vi "Start GNU Octave.vi"(0 "working dir (user home)":path, 1 "full start timeout [ms] (20000)":u32=20000, 2 "Matlab script mode (F)":bool, 5 "octave binary file or dir (autofind)":path, 7 "path to lv_proc.dll (.)":path, 9 "hide debug console (T)":bool=TRUE, 11 "error in":errorcluster, 12 "wait for full start (T)":bool=TRUE, 13 "disable history (T)":bool=TRUE) -> (3 "GNU Octave version":string, 4 "GOLPI ref. out":T1={"pipe handle"={"lv_proc.dll file path"=path "", "process instance handle"=[], "debug mode"=FALSE, "debug data"=[]}, "fast read timeout [ms]"=500, "fast read settle time [ms]"=10, "fast read to multiple [ms]"=1, "max elements per input line"=100, "slow read timeout [ms]"=500, "stdin double format specifier"="", "max elements per stdout output column"=100, "console mode bitstream"=FALSE, "bitstream first read timeout [ms]"=1000, "bitstream read timeout [ms]"=50, "struct transfer possible"=FALSE, "matlab mode"=FALSE, "var pipe write timeout [ms]"=5000, "variable pipe mode"=FALSE, "variable pipe buffer size [Bytes]"=10000000, "variable pipe block size [Bytes]"=1000000} {"variable pipe block size [Bytes]" format="%.0p"; "variable pipe buffer size [Bytes]" format="%.0p"}, 14 "initial output":string, 15 "error out":errorcluster)   [LabVIEW 2020, in "GOLPI library.lvlib"]
doc: "Starts the GNU Octave.\nIf working directory is empty, VI sets it to user Documents directory.\n\nOctave binary file or directory is the executable file or directory containing the 'octave.bat' executable file (or 'octave-cli.exe', 'octave.exe'). Script .bat is prefered, because it sets libraries paths properly. If ommited, VI tries to find latest Octave installation.\n\nInitial output is the informations printed after start on the screen by GNU Octave. Set higher vlaue for 'Full start timeout' in the case GNU Octave loads a lot of packages.\n\nIf option 'Matlab script mode' is True, the VI will start Matlab using NI's Matlab script node. All followed VI calls of this library will then use Matlab instead of GNU Octave. That also means only used input option is 'wait fo full start'. Rest will be ignored.\n\nIf 'Wait for full start' is disabled, vi starts GNU Octave/Matlab and do not wait for the end of starting sequence. It is usefull if GNU Octave/Matlab loads a lot of packages at startup and the start can take several seconds. 'Version' and 'Initial output' is not returned. User can check himself if Octave finished starting sequence by waiting for keyword 'GOLPImarkstart' in the stdout (i.e. use 'Read Output Till Keyword.vi'). Note this is not supported for Matlab mode.\n\nSet 'hide window' to false to show console window (no effect in Matlab mode). Thus user can watch commands sent to GNU Octave and its output. Window is not interactive, only for debug purposes.\n\nIf 'Disable history' is set, all commands sent to GNU Octave will not be saved to GNU Octave history file. This is recommended especially when large data transfers are expected. This has no effect in Matlab mode.\n\n---\nGOLPI works only with 'lv_proc.dll' library in the GNU Octave mode, which is part of vipm package or should be delivered together with packed library. Placement of this dll is selected in terminal of Start GNU Octave.vi."
uses:
  GOLPI library.lvlib
  GOLPI reference Type Def.ctl
  LV Process source distribution/Pipe Handle.ctl
  <vilib>/Utility/sysdir.llb/System Directory Type.ctl
  Private/Type Definitions/Custom Error Codes Enum Type Def.vi
  <vilib>/regexp/Match Regular Expression.xnode
  LV Process source distribution/LV Process library.lvlib
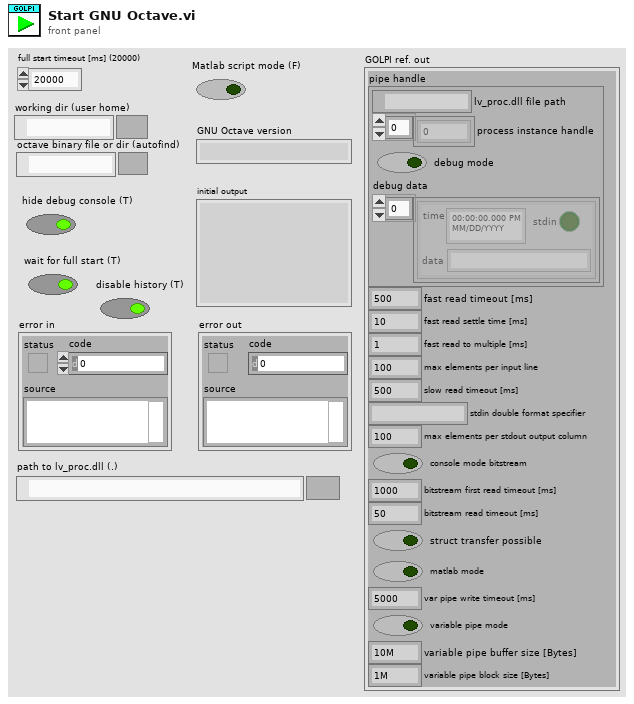
[diagram p1: front panel]
types:
  T1 = typedef "GOLPI library.lvlib/GOLPI reference Type Def.ctl" = cluster{"pipe handle":T2, "fast read timeout [ms]":u32, "fast read settle time [ms]":u32, "fast read to multiple [ms]":u32, "max elements per input line":u32, "slow read timeout [ms]":u32, "stdin double format specifier":string, "max elements per stdout output column":u32, "console mode bitstream":bool, "bitstream first read timeout [ms]":u32, "bitstream read timeout [ms]":u32, "struct transfer possible":bool, "matlab mode":bool, "var pipe write timeout [ms]":u32, "variable pipe mode":bool, "variable pipe buffer size [Bytes]":u32, "variable pipe block size [Bytes]":u32}
  T2 = typedef "LV Process library.lvlib/Pipe Handle.ctl" = cluster{"lv_proc.dll file path":path, "process instance handle":u32[], "debug mode":bool, "debug data":cluster{"time":timestamp, "stdin":bool, "data":string}[]}
  T3 = typedef "GOLPI library.lvlib/Custom Error Codes Enum Type Def.vi" = enum16{"no error", "00 working directory PAR1 missing", "01 octave binary PAR1 missing", "02 octave report error PAR1", "03 empty output last cmd PAR1", "04 missing temporary file PAR1", "05 pwd PAR 1 not exist", "06 oct package not installed", "07 octave default binary missing", "10 var PAR1 not string, vect", "11 var PAR1 not num, scal, ~compl", "12 var PAR1 not num, scal, compl", "13 var PAR1 not num, vect, ~compl", "14 var PAR1 not num, vect, compl", "15 var PAR1 not num, mat, ~compl", "16 var PAR1 not num, mat, ~compl", "30 read timeout", "60 bitstream transport failed", "61 bitstream decode error PAR1", "62 bitstream cannot be set", "70 struct transfer not possible", "80 struct: cluster elem. PAR1 not implem.", "81 struct: structure field PAR1 not implem.", "82 struct: size mismatch of PAR1", "83 struct: type mismatch of PAR1", "98 internal error", "99 not finished", "90 Not supported in Matlab mode", "91 Matlab variable transfer error", "92 Matlab Script Error", "100 Variable Pipe Mode cannot be set"}
  T4 = typedef "System Directory Type.ctl" = i32
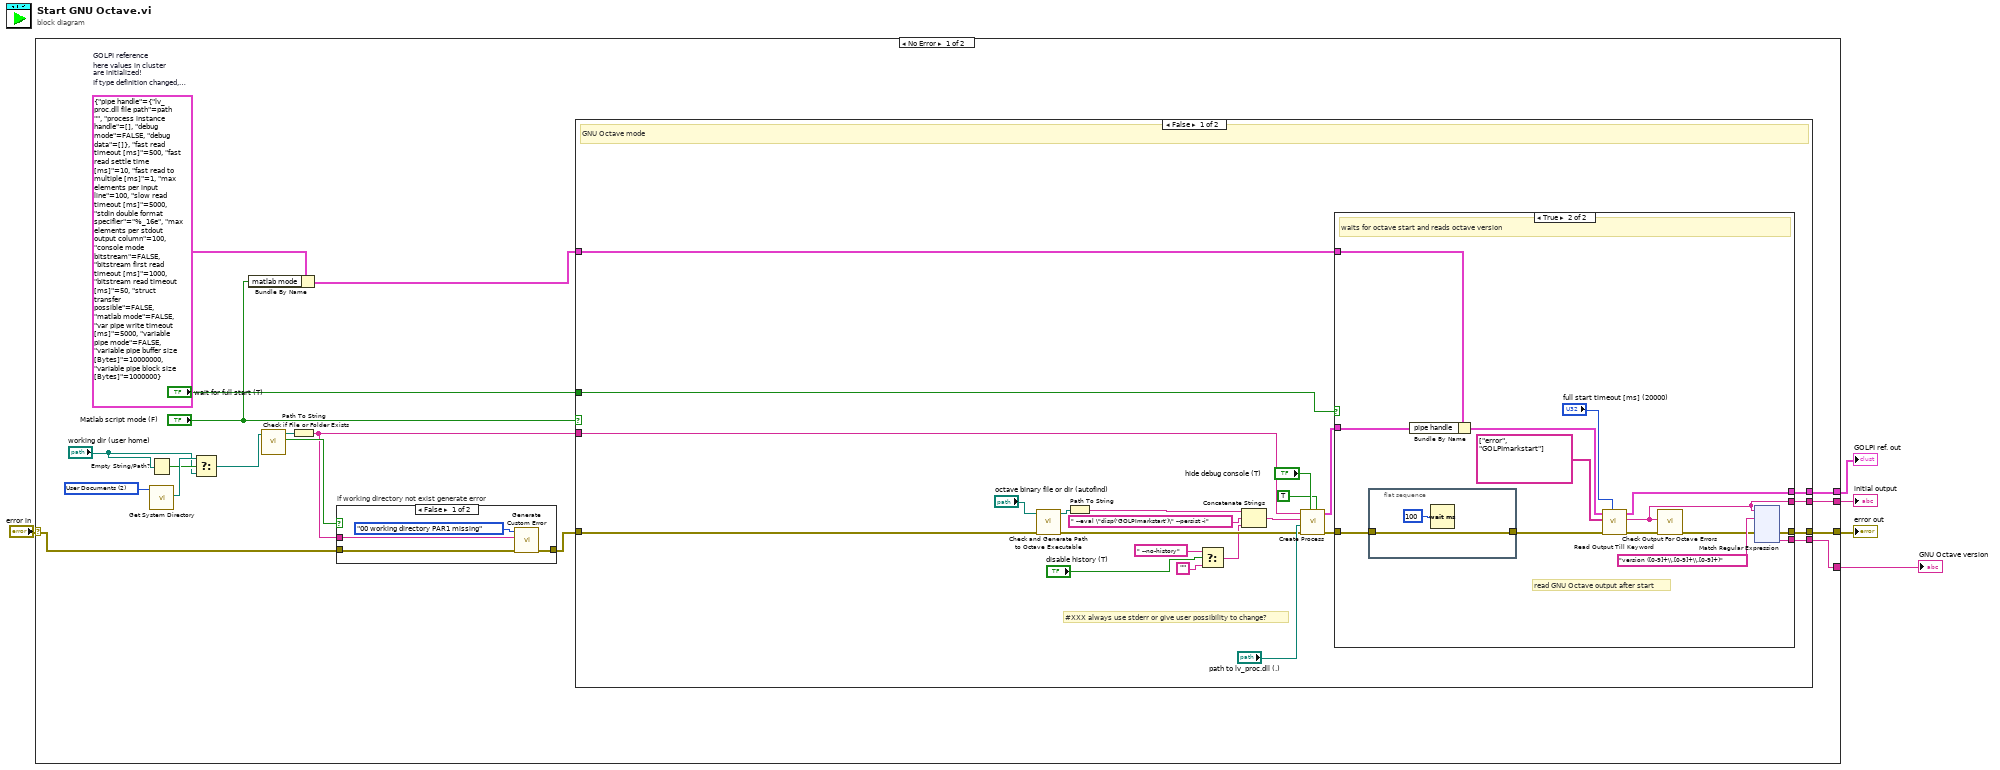
[diagram p0: block diagram]
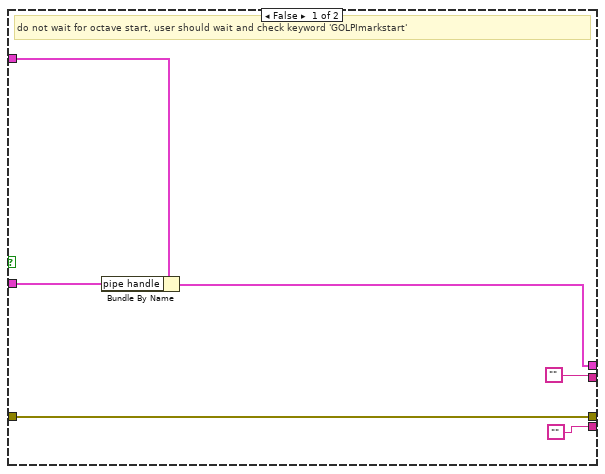
[diagram p3: hidden frame]
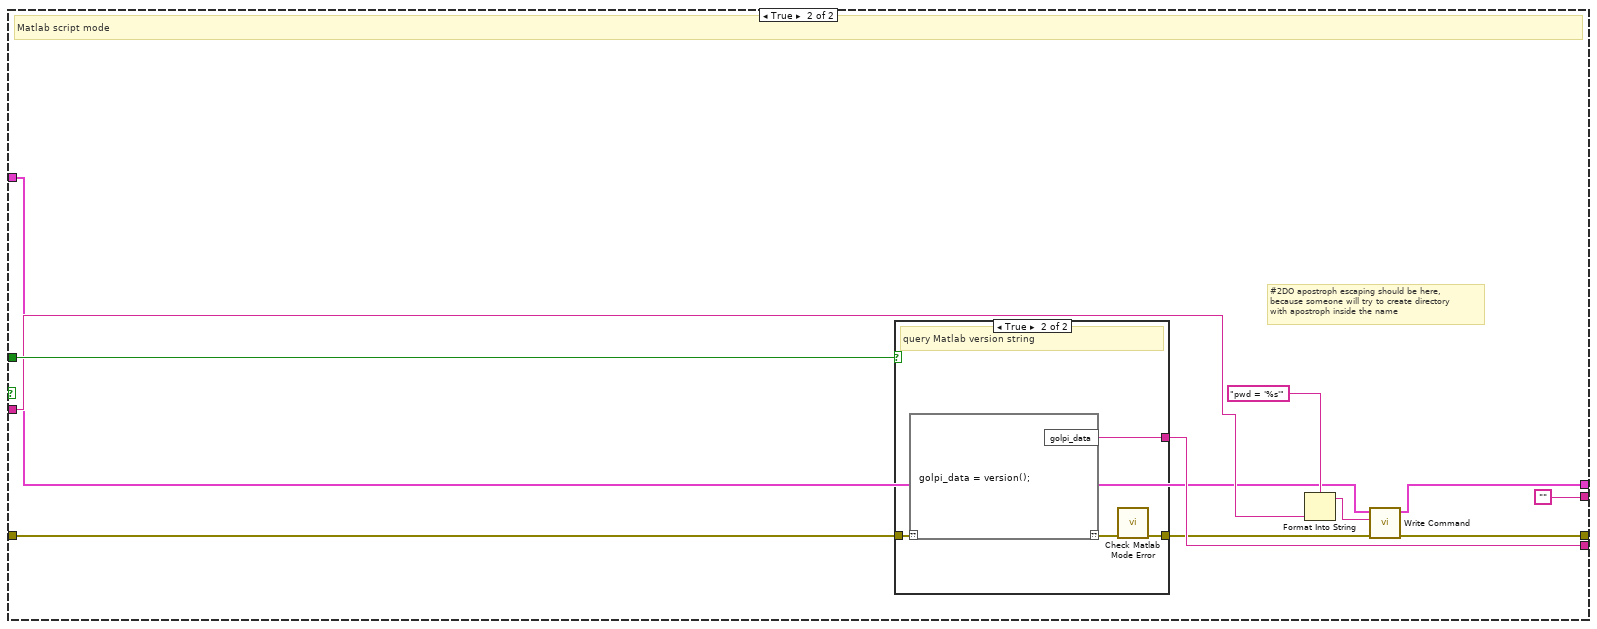
[diagram p4: hidden frame]
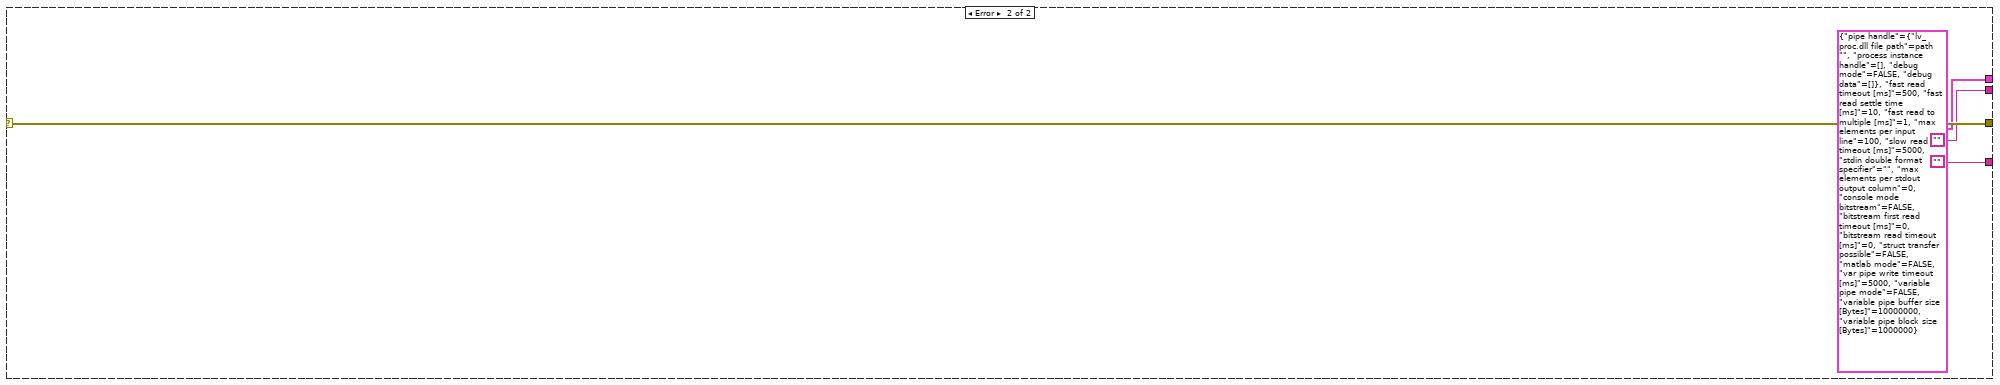
[diagram p6: hidden frame]
diagram:
  n1 = case shown="No Error" "error in" {
    selector: "error in" -> [w6 w209]
    tunnel: [w21 w209] -> w4
    tunnel: [w23 ""] -> w3
    tunnel: [w20 ""] -> w2
    tunnel: [w22 T1 {"pipe handle"={"lv_proc.dll file path"=path "", "process instance handle"=[], "debug mode"=FALSE, "debug data"=[]}, "fast read timeout [ms]"=500, "fast read settle time [ms]"=10, "fast read to multiple [ms]"=1, "max elements per input line"=100, "slow read timeout [ms]"=5000, "stdin double format specifier"="", "max elements per stdout output column"=0, "console mode bitstream"=FALSE, "bitstream first read timeout [ms]"=0, "bitstream read timeout [ms]"=0, "struct transfer possible"=FALSE, "matlab mode"=FALSE, "var pipe write timeout [ms]"=5000, "variable pipe mode"=FALSE, "variable pipe buffer size [Bytes]"=10000000, "variable pipe block size [Bytes]"=1000000} ("GOLPI ref.")] -> w1
    frame No Error {
      w15 = T4 2 items=["User Home"=0, "User Desktop"=1, "User Documents"=2, "User Application Data"=3, "User Preferences"=4, "User Temporary"=5, "Public Documents"=6, "Public Application Data"=7, "Public Preferences"=8, "Public Cache"=13, "System Core Libraries"=9, "System Installed Libraries"=10, "Application Files"=11, "Boot Volume Root"=12] ("system directory type")
      w18 = T1 {"pipe handle"={"lv_proc.dll file path"=path "", "process instance handle"=[], "debug mode"=FALSE, "debug data"=[]}, "fast read timeout [ms]"=500, "fast read settle time [ms]"=10, "fast read to multiple [ms]"=1, "max elements per input line"=100, "slow read timeout [ms]"=5000, "stdin double format specifier"="%_16e", "max elements per stdout output column"=100, "console mode bitstream"=FALSE, "bitstream first read timeout [ms]"=1000, "bitstream read timeout [ms]"=50, "struct transfer possible"=FALSE, "matlab mode"=FALSE, "var pipe write timeout [ms]"=5000, "variable pipe mode"=FALSE, "variable pipe buffer size [Bytes]"=10000000, "variable pipe block size [Bytes]"=1000000}  # GOLPI reference here values in cluster are initialized! If type definition changed, values here have to be updated!
      n2 = Empty String/Path?(string/path="working dir (user home)") -> (empty?=w13:bool)
      n3 = call <vilib>:"Get System Directory.vi"("system directory type"=w15) -> ("system directory"=w14:path)  [unwired: 10 in]
      n4 = Select(t=w14, s=w13, f="working dir (user home)") -> (s? t:f=w7:path)
      n5 = Bundle By Name(cluster=w18, "matlab mode"="Matlab script mode (F)") -> (w17:T1)
      n6 = call <vilib>:"Check if File or Folder Exists.vi"("path"=w7) -> ("file or folder exists?"=w11:bool, "dup path"=w10:path)  [unwired: 8 in, 1 out]
      n7 = Path To String(path=w10) -> (string=w8:string)
      n8 = case "if working directory not exist generate error" shown="False" w11 {
        tunnel: [w25 w28] -> w9
        tunnel: w6 -> [w24 w28]
        tunnel: w8 -> [w27 _]
        frame False {
          n9 = call "Generate Custom Error.vi"("error in"=w24, "PAR1"=w27, "GOLPI error"=Custom_Error_Codes_Enum_Type_Def.vi."00 working directory PAR1 missing" ("Enum")) -> ("error out"=w25:errorcluster)  [unwired: 8 in]
        }
        frame True {
        }
      }
      n10 = case shown="False" "Matlab script mode (F)" {
        tunnel: w9 -> [w30 w200]
        tunnel: [w48 w199] -> w23
        tunnel: w17 -> [w47 w192]
        tunnel: [w45 w191] -> w22
        tunnel: [w41 w196] -> w21
        tunnel: [w40 ""] -> w20
        tunnel: "wait for full start (T)" -> [w39 w198]
        tunnel: w8 -> [w29 w194]
        frame False {
          # "#XXX always use stderr or give user possibility to change?"
          # "GNU Octave mode"
          n11 = call "Check and Generate Path to Octave Executable.vi"("error in (no error)"=w30, "octave executable file or directory with executable"="octave binary file or dir (autofind)") -> ("error out"=w37:errorcluster, "path to exe"=w35:path)  [unwired: 8 in]
          n12 = Path To String(path=w35) -> (string=w44:string)
          n13 = Select(t=" --no-history" ("string"), s="disable history (T)", f="") -> (s? t:f=w32:string)
          n14 = Concatenate Strings(w44, " --eval \"disp('GOLPImarkstart')\" --persist -i" ("string"), w32) -> (w42:string)
          n15 = call "Create Process.vi"("use stderr (F)"=TRUE, "hide window (T)"="hide debug console (T)", "error in"=w37, "dir or path to lv_proc.dll (.)"="path to lv_proc.dll (.)", "command"=w42, "working directory"=w29) -> ("error out"=w49:errorcluster, "pipe out"=w46:T2)  [unwired: 4 in]
          n16 = case shown="True" w39 {
            tunnel: w49 -> [w57 w71]
            tunnel: ["" w68] -> w48
            tunnel: w47 -> [w54 w67]
            tunnel: w46 -> [w53 w66]
            tunnel: [w52 w64] -> w45
            tunnel: [w57 w63] -> w41
            tunnel: ["" w59] -> w40
            frame False {
              # "do not wait for octave start, user should wait and check keyword 'GOLPImarkstart'"
              n17 = Bundle By Name(cluster=w54, "pipe handle"=w53) -> (w52:T1)
            }
            frame True {
              # "read GNU Octave output after start"
              # "waits for octave start and reads octave version"
              n18 = flat-sequence {
                tunnel: [w188] -> w70
                tunnel: w71 -> [w188]
                frame #0 {
                  n19 = Wait (ms)(milliseconds to wait=u32 100) -> ()  [unwired: 1 out]
                }
              }
              n20 = Bundle By Name(cluster=w67, "pipe handle"=w66) -> (w65:T1)
              n21 = call "Read Output Till Keyword.vi"("timeout [ms]"="full start timeout [ms] (20000)", "error in"=w70, "keywords"=string[] ["error", "GOLPImarkstart"], "GOLPI ref. in"=w65) -> ("error out"=w61:errorcluster, "read buffer"=w59:string, "GOLPI ref. out"=w64:T1)  [unwired: 4 in, 1 out]
              n22 = call "Check Output For Octave Errors.vi"("error in"=w61, "read buffer"=w59) -> ("error out"=w60:errorcluster)  [unwired: 9 in]
              n23 = xnode "Match Regular Expression"("input string"=w59, "regular expression"="version ([0-9]+\\.[0-9]+\\.[0-9]+)", "error in"=w60) -> ("error out"=w63:errorcluster, "submatch 1"=w68:string)  [unwired: 3 in, 4 out]
            }
          }
        }
        frame True {
          # "#2DO apostroph escaping should be here,\nbecause someone will try to create directory\nwith apostroph inside the name"
          # "Matlab script mode"
          n24 = case shown="True" w198 {
            tunnel: w200 -> [w201 w205]
            tunnel: [w201 w202] -> w197
            tunnel: [_ w204] -> w199
            frame False {
              # "do not wait"
            }
            frame True {
              # "query Matlab version string"
              n25 = script code="golpi_data = version();"("??"=w205) -> ("??"=w203:errorcluster, "golpi_data"=w204:string)
              n26 = call "Check Matlab Mode Error.vi"("error in"=w203) -> ("error out"=w202:errorcluster)  [unwired: 10 in]
            }
          }
          n27 = Format Into String(format string="pwd = '%s'", w194) -> (resulting string=w193:string)  [unwired: 2 in, 1 out]
          n28 = call "Write Command.vi"("error in"=w197, "command"=w193, "GOLPI ref. in"=w192) -> ("error out"=w196:errorcluster, "GOLPI ref. out"=w191:T1)  [unwired: 7 in]
        }
      }
    }
    frame Error {
    }
  }
  "error out" <- w4
  "GNU Octave version" <- w3
  "initial output" <- w2
  "GOLPI ref. out" <- w1
